vi "str_R_SWING.vi"() -> ()   [LabVIEW 2015]
uses:
  <vilib>/NXT/Subs/MotorOutput.ctl
  <vilib>/NXT/Block Support/NXT_InputPort.ctl
  <vilib>/NXT/Dual Mode Library/Motors/MotorBrake.vi
  <vilib>/NXT/Dual Mode Library/Motors/MotorOn.vi
  <vilib>/NXT/Dual Mode Library/Waits/Wait_Num.vi
  <vilib>/NXT/Dual Mode Library/Sensors/Light_On.vi
  <vilib>/NXT/Dual Mode Library/Sensors/Sonar_cm.vi
  <vilib>/NXT/Dual Mode Library/Motors/MotorReverse.vi
  <vilib>/NXT/Dual Mode Library/Motors/MotorCoast.vi
panel:
  in  "stop":bool
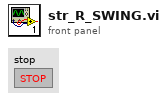
[diagram p1: front panel]
types:
  T1 = typedef "MotorOutput.ctl" = u8
  T2 = typedef "LVHSConnector.ctl" = refnum<class "BrickReference.lvclass">
  T3 = typedef "NXT_InputPort.ctl" = u32
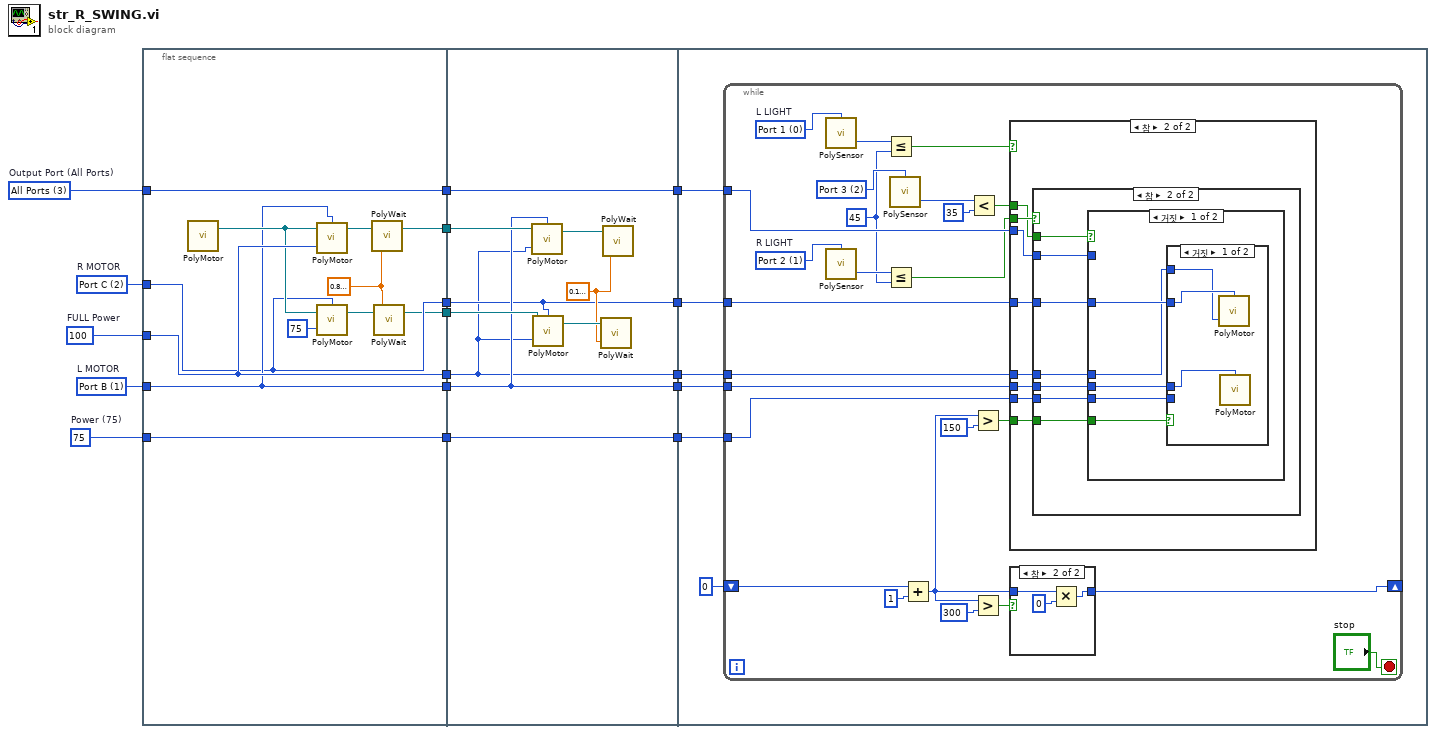
[diagram p0: block diagram]
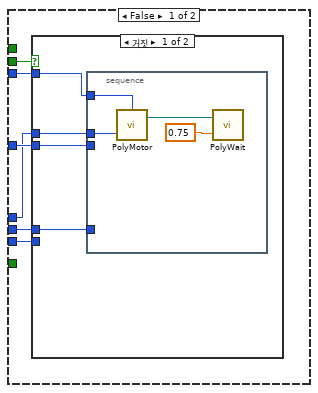
[diagram p3: hidden frame]
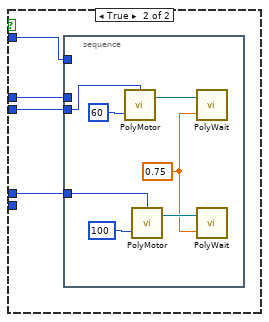
[diagram p4: hidden frame]
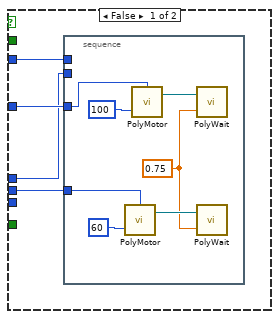
[diagram p5: hidden frame]
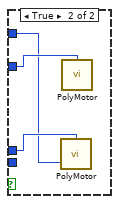
[diagram p6: hidden frame]
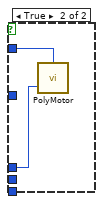
[diagram p7: hidden frame]
diagram:
  w13 = 100  # FULL Power
  w14 = 75  # Power (75)
  w15 = T1 2 items=["Port A"=0, "Port B"=1, "Port C"=2, "Ports A & B"=4, "Ports A & C"=5, "Ports B & C"=6, "All Ports"=3]  # R MOTOR
  w16 = T1 1 items=["Port A"=0, "Port B"=1, "Port C"=2, "Ports A & B"=4, "Ports A & C"=5, "Ports B & C"=6, "All Ports"=3]  # L MOTOR
  w17 = T1 3 items=["Port A"=0, "Port B"=1, "Port C"=2, "Ports A & B"=4, "Ports A & C"=5, "Ports B & C"=6, "All Ports"=3]  # Output Port (All Ports)
  n1 = flat-sequence {
    tunnel: w17 -> [w29]
    tunnel: w16 -> [w22]
    tunnel: w15 -> [w21]
    tunnel: w14 -> [w23]
    tunnel: w13 -> [w27]
    tunnel: [w29] -> w12
    tunnel: [w22] -> w10
    tunnel: [w21] -> w8
    tunnel: [w23] -> w6
    tunnel: [w27] -> w4
    tunnel: [w20] -> w2
    tunnel: [w19] -> w1
    tunnel: w12 -> [w38]
    tunnel: [w38] -> w11
    tunnel: w10 -> [w32]
    tunnel: [w32] -> w9
    tunnel: w8 -> [w31]
    tunnel: [w31] -> w7
    tunnel: w6 -> [w39]
    tunnel: [w39] -> w5
    tunnel: w4 -> [w30]
    tunnel: [w30] -> w3
    tunnel: w2 -> [w36]
    tunnel: w1 -> [w35]
    tunnel: w11 -> [w45]
    tunnel: w9 -> [w44]
    tunnel: w7 -> [w43]
    tunnel: w5 -> [w42]
    tunnel: w3 -> [w41]
    frame #0 {
      w26 = sgl 0.8 ("Time (1 sec)")
      n2 = call-poly <vilib>:"PolyMotor.vi"() -> ("NXT/EV3"=w24:T2)  [unwired: 2 in, 2 out]
      n3 = call-poly <vilib>:"PolyMotor.vi"("Power (75)"=w27, "NXT/EV3"=w24, "Output Port (All Ports)"=w22) -> ("NXT/EV3"=w28:T2)  [unwired: 1 out]
      n4 = call-poly <vilib>:"PolyMotor.vi"("Power (75)"=75, "NXT/EV3"=w24, "Output Port (All Ports)"=w21) -> ("NXT/EV3"=w25:T2)  [unwired: 1 out]
      n5 = call-poly <vilib>:"PolyWait.vi"("Time (1 sec)"=w26, "NXT/EV3"=w28) -> ("NXT/EV3"=w20:T2)  [unwired: 2 in]
      n6 = call-poly <vilib>:"PolyWait.vi"("Time (1 sec)"=w26, "NXT/EV3"=w25) -> ("NXT/EV3"=w19:T2)  [unwired: 2 in]
    }
    frame #1 {
      w33 = sgl 0.1 ("Time (1 sec)")
      n7 = call-poly <vilib>:"PolyMotor.vi"("Power (75)"=w30, "NXT/EV3"=w36, "Output Port (All Ports)"=w32) -> ("NXT/EV3"=w37:T2)  [unwired: 1 out]
      n8 = call-poly <vilib>:"PolyMotor.vi"("Power (75)"=w30, "NXT/EV3"=w35, "Output Port (All Ports)"=w31) -> ("NXT/EV3"=w34:T2)  [unwired: 1 out]
      n9 = call-poly <vilib>:"PolyWait.vi"("Time (1 sec)"=w33, "NXT/EV3"=w34) -> ()  [unwired: 2 in, 1 out]
      n10 = call-poly <vilib>:"PolyWait.vi"("Time (1 sec)"=w33, "NXT/EV3"=w37) -> ()  [unwired: 2 in, 1 out]
    }
    frame #2 {
      n11 = while {
        tunnel: w45 -> [w65]
        tunnel: w44 -> [w64]
        tunnel: w43 -> [w63]
        tunnel: w42 -> [w62]
        tunnel: w41 -> [w61]
        shift-right: [w48] -> _
        shift-left: i16 0 ("y") -> [w56]
        stop <- "stop" stop-if-true
        w60 = T3 2 items=["Port 1", "Port 2", "Port 3", "Port 4"] ("Port (Port 4)")
        w66 = T3 1 items=["Port 1", "Port 2", "Port 3", "Port 4"]  # R LIGHT
        w69 = T3 0 items=["Port 1", "Port 2", "Port 3", "Port 4"]  # L LIGHT
        w49 = i16 45 ("Scaled Value")
        n12 = call-poly <vilib>:"PolySensor.vi"("Port (Port 3)"=w69) -> ("Scaled Value"=w68:i16)  [unwired: 2 in, 1 out]
        n13 = call-poly <vilib>:"PolySensor.vi"("Port (Port 3)"=w66) -> ("Scaled Value"=w67:i16)  [unwired: 2 in, 1 out]
        n14 = Less Or Equal?(x=w68, y=w49) -> (x <= y?=w47:bool)
        n15 = Less Or Equal?(x=w67, y=w49) -> (x <= y?=w46:bool)
        n16 = call-poly <vilib>:"PolySensor.vi"("Port (Port 4)"=w60) -> ("Distance (cm)"=w59:i16)  [unwired: 2 in, 1 out]
        n17 = Add(x=w56, y=i16 1) -> (x+y=w50:i16)
        n18 = Less?(x=w59, y=i16 35) -> (x < y?=w57:bool)
        n19 = Greater?(x=w50, y=i16 150) -> (0:w52:bool)
        n20 = Greater?(x=w50, y=i16 300) -> (0:w55:bool)
        n21 = case shown="참" w47 {
          tunnel: w65 -> [w79 w107]
          tunnel: w62 -> [w78 w106]
          tunnel: w46 -> [w80 w102]
          tunnel: w63 -> [w77 w104]
          tunnel: w64 -> [w76 w105]
          tunnel: w61 -> [w75 w103]
          tunnel: w57 -> [_ w101]
          tunnel: w52 -> [_ w100]
          frame False {
            n22 = case shown="거짓" w80 {
              tunnel: w79 -> [w84 w89]
              tunnel: w78 -> [_ _]
              tunnel: w76 -> [w82 w92]
              tunnel: w77 -> [w81 w91]
              tunnel: w75 -> [w83 w90]
              frame False {
                n23 = stacked-sequence {
                  tunnel: w84 -> [w88]
                  tunnel: w83 -> [w85]
                  tunnel: w82 -> [_]
                  tunnel: w81 -> [_]
                  frame #0 {
                    n24 = call-poly <vilib>:"PolyMotor.vi"("Power (75)"=w85, "Output Port (All Ports)"=w88) -> ("NXT/EV3"=w87:T2)  [unwired: 1 in, 1 out]
                    n25 = call-poly <vilib>:"PolyWait.vi"("Time (1 sec)"=sgl 0.75, "NXT/EV3"=w87) -> ()  [unwired: 2 in, 1 out]
                  }
                }
              }
              frame True {
                n26 = stacked-sequence {
                  tunnel: w92 -> [w95]
                  tunnel: w91 -> [w94]
                  tunnel: w90 -> [_]
                  tunnel: w89 -> [_]
                  frame #0 {
                    w93 = sgl 0.75 ("Time (1 sec)")
                    n27 = call-poly <vilib>:"PolyMotor.vi"("Power (75)"=60 ("Power (75) 5"), "Output Port (All Ports)"=w94) -> ("NXT/EV3"=w96:T2)  [unwired: 1 in, 1 out]
                    n28 = call-poly <vilib>:"PolyMotor.vi"("Power (75)"=100 ("Power (75) 4"), "Output Port (All Ports)"=w95) -> ("NXT/EV3"=w97:T2)  [unwired: 1 in, 1 out]
                    n29 = call-poly <vilib>:"PolyWait.vi"("Time (1 sec)"=w93, "NXT/EV3"=w96) -> ()  [unwired: 2 in, 1 out]
                    n30 = call-poly <vilib>:"PolyWait.vi"("Time (1 sec)"=w93, "NXT/EV3"=w97) -> ()  [unwired: 2 in, 1 out]
                  }
                }
              }
            }
          }
          frame True {
            n31 = case shown="참" w102 {
              tunnel: w107 -> [w109 w125]
              tunnel: w106 -> [_ w122]
              tunnel: w105 -> [w111 w121]
              tunnel: w104 -> [w110 w120]
              tunnel: w103 -> [w108 w124]
              tunnel: w101 -> [_ w123]
              tunnel: w100 -> [_ w119]
              frame False {
                n32 = stacked-sequence {
                  tunnel: w111 -> [w116]
                  tunnel: w110 -> [w112]
                  tunnel: w109 -> [_]
                  tunnel: w108 -> [_]
                  frame #0 {
                    w113 = sgl 0.75 ("Time (1 sec)")
                    n33 = call-poly <vilib>:"PolyMotor.vi"("Power (75)"=60 ("Power (75) 2"), "Output Port (All Ports)"=w116) -> ("NXT/EV3"=w114:T2)  [unwired: 1 in, 1 out]
                    n34 = call-poly <vilib>:"PolyMotor.vi"("Power (75)"=100 ("Power (75) 3"), "Output Port (All Ports)"=w112) -> ("NXT/EV3"=w117:T2)  [unwired: 1 in, 1 out]
                    n35 = call-poly <vilib>:"PolyWait.vi"("Time (1 sec)"=w113, "NXT/EV3"=w117) -> ()  [unwired: 2 in, 1 out]
                    n36 = call-poly <vilib>:"PolyWait.vi"("Time (1 sec)"=w113, "NXT/EV3"=w114) -> ()  [unwired: 2 in, 1 out]
                  }
                }
              }
              frame True {
                n37 = case shown="거짓" w123 {
                  tunnel: w125 -> [_ w138]
                  tunnel: w124 -> [w126 w137]
                  tunnel: w122 -> [w130 _]
                  tunnel: w121 -> [w129 _]
                  tunnel: w120 -> [w128 _]
                  tunnel: w119 -> [w127 _]
                  frame False {
                    n38 = case shown="거짓" w127 {
                      tunnel: w130 -> [_ _]
                      tunnel: w129 -> [w133 w136]
                      tunnel: w128 -> [w132 w135]
                      tunnel: w126 -> [w131 w134]
                      frame False {
                        n39 = call-poly <vilib>:"PolyMotor.vi"("Power (75)"=w131, "Output Port (All Ports)"=w132) -> ()  [unwired: 1 in, 2 out]
                        n40 = call-poly <vilib>:"PolyMotor.vi"("Port (All Ports)"=w133) -> ()  [unwired: 1 in, 3 out]
                      }
                      frame True {
                        n41 = call-poly <vilib>:"PolyMotor.vi"("Power (75)"=w134, "Output Port (All Ports)"=w136) -> ()  [unwired: 1 in, 2 out]
                        n42 = call-poly <vilib>:"PolyMotor.vi"("Port (All Ports)"=w135) -> ()  [unwired: 1 in, 3 out]
                      }
                    }
                  }
                  frame True {
                    n43 = call-poly <vilib>:"PolyMotor.vi"("Power (75)"=w137, "Output Port (All Ports)"=w138) -> ()  [unwired: 1 in, 2 out]
                  }
                }
              }
            }
          }
        }
        n44 = case shown="참" w55 {
          tunnel: w50 -> [w71 w74]
          tunnel: [w71 w72] -> w48
          frame False {
          }
          frame True {
            n45 = Multiply(x=w74, y=i16 0) -> (x*y=w72:i16)
          }
        }
      }
    }
  }
